vi "Is Complete.vi"(8 "error in (no error)":errorcluster, 11 "Operation Complete Caller in":refnum<class "Operation Complete Caller.lvclass">) -> (0 "error out":errorcluster, 2 "Complete":bool, 3 "Operation Complete Caller out":refnum<class "Operation Complete Caller.lvclass">)   [LabVIEW 2022 SP3, in "Operation Complete Caller.lvclass"]
uses:
  Operation Complete Caller.lvclass
  Operation Complete Caller.lvclass/Operation Complete Caller.ctl
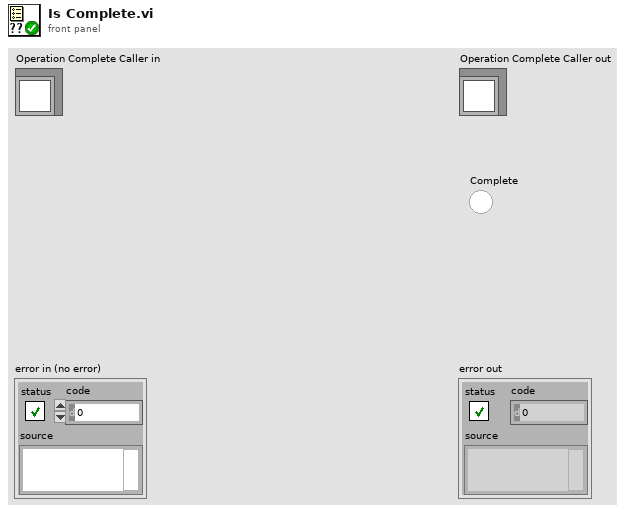
[diagram p1: front panel]
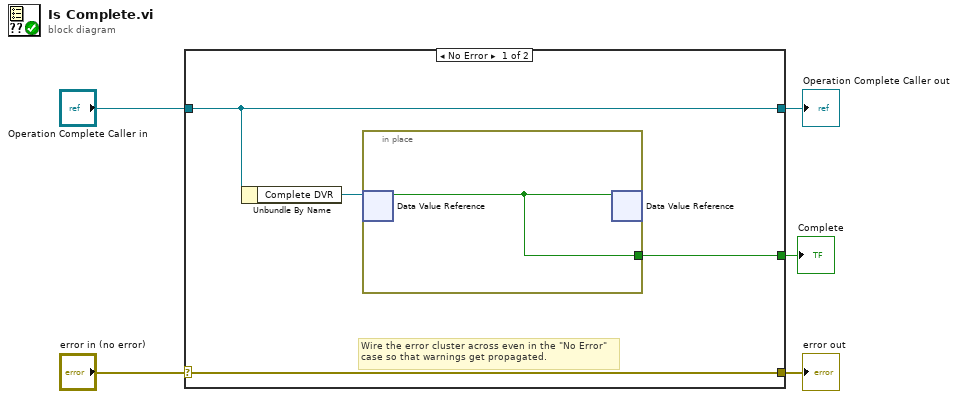
[diagram p0: block diagram]
diagram:
  n1 = case shown="No Error" "error in (no error)" {
    selector: "error in (no error)" -> [w9 w12]
    tunnel: [w9 w12] -> w4
    tunnel: [w8 w11] -> w2
    tunnel: "Operation Complete Caller in" -> [w8 w11]
    tunnel: [w6 _] -> w1
    frame No Error {
      # "Wire the error cluster across even in the \"No Error\"\ncase so that warnings get propagated."
      n2 = Unbundle By Name(w8) -> ("Complete DVR"=w7:refnum<data-value>)
      n3 = in-place {
        in-place-border: [w10] -> w6
        n4 = in-place-dvr #1(w7) -> (w10:bool)  [unwired: 1 out]
        n5 = in-place-dvr #1(w10) -> ()  [unwired: 2 out]
      }
    }
    frame Error {
    }
  }
  "error out" <- w4
  "Operation Complete Caller out" <- w2
  "Complete" <- w1
